vi "Simulation-07.vi"() -> ()   [LabVIEW 2020]
uses:
  librarian_class/typedefs/book_state--enum.ctl
  shared/request--enum.ctl
  librarian_class/librarian.lvclass
  client_class/client.lvclass
panel:
  out "success":bool
  out "lib error out":errorcluster
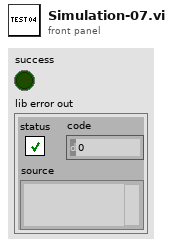
[diagram p1: front panel]
types:
  T1 = typedef "request--enum.ctl" = enum16{"CHECKIN", "CHECKOUT"}
  T2 = typedef "librarian.lvclass/book_state--enum.ctl" = enum16{"CHECKEDIN", "CHECKEDOUT", "DAMAGED"}
  T3 = typedef "message--cluster.ctl" = cluster{"header":string, "cmd":T1, "title":string, "book":string}
  T4 = typedef "librarian.lvclass/lib_map_value--cluster.ctl" = cluster{"book state":T2, "text":string, "hash":string}
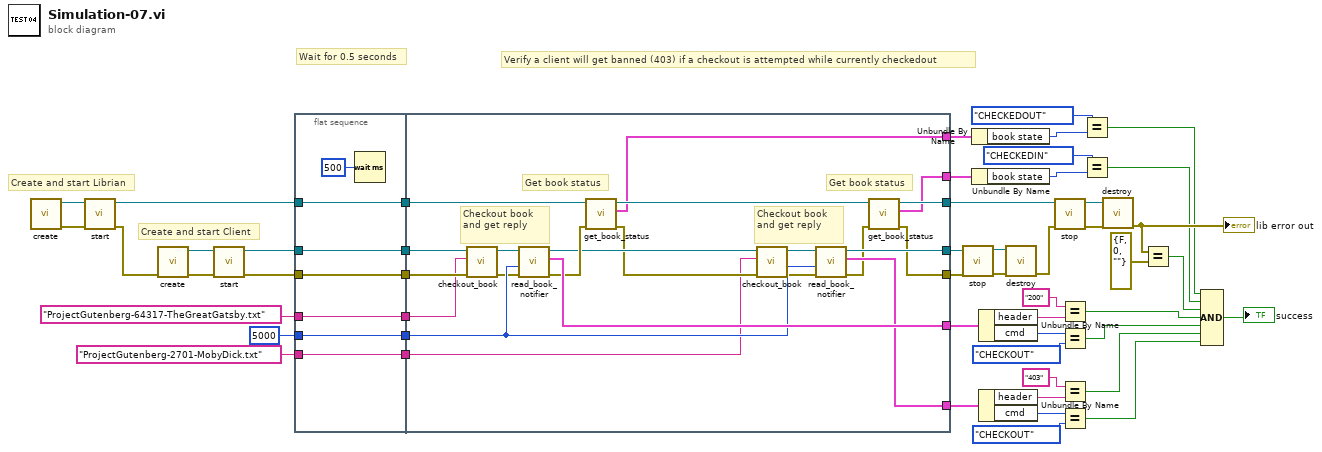
[diagram p0: block diagram]
diagram:
  # "Verify a client will get banned (403) if a checkout is attempted while currently checkedout"
  # "Wait for 0.5 seconds"
  # "Create and start Client"
  # "Create and start Librian"
  n1 = call "create.vi"() -> ("error out"=w50:errorcluster, "librarian_sm out"=w51:refnum<class "librarian.lvclass">)  [unwired: 10 in]
  n2 = call "start.vi"("error in (no error)"=w50, "librarian_sm in"=w51) -> ("error out"=w30:errorcluster, "librarian_sm out"=w41:refnum<class "librarian.lvclass">)  [unwired: 8 in]
  n3 = call "create.vi"("error in (no error)"=w30) -> ("error out"=w46:errorcluster, "librarian_sm out"=w47:refnum<class "client.lvclass">)  [unwired: 9 in]
  n4 = call "start.vi"("error in (no error)"=w46, "librarian_sm in"=w47) -> ("error out"=w43:errorcluster, "librarian_sm out"=w42:refnum<class "client.lvclass">)  [unwired: 8 in]
  n5 = flat-sequence {
    tunnel: "ProjectGutenberg-64317-TheGreatGatsby.txt" ("book title") -> [w53]
    tunnel: 5000 ("timeout in ms (-1)") -> [w56]
    tunnel: w41 -> [w57]
    tunnel: w42 -> [w58]
    tunnel: w43 -> [w54]
    tunnel: [w54] -> w35
    tunnel: [w58] -> w34
    tunnel: [w57] -> w33
    tunnel: [w56] -> w32
    tunnel: [w53] -> w31
    tunnel: [w52] -> w2
    tunnel: "ProjectGutenberg-2701-MobyDick.txt" ("book title") -> [w52]
    tunnel: [w80] -> w14
    tunnel: [w67] -> w38
    tunnel: [w78] -> w39
    tunnel: [w70] -> w40
    tunnel: [w77] -> w13
    tunnel: w31 -> [w61]
    tunnel: w32 -> [w79]
    tunnel: w33 -> [w72]
    tunnel: w34 -> [w75]
    tunnel: w35 -> [w76]
    tunnel: [w66] -> w23
    tunnel: [w65] -> w24
    tunnel: w2 -> [w59]
    frame #0 {
      n6 = Wait (ms)(milliseconds to wait=u32 500) -> ()  [unwired: 1 out]
    }
    frame #1 {
      # "Get book status"
      # "Get book status"
      # "Checkout book and get reply"
      # "Checkout book and get reply"
      n7 = call "checkout_book.vi"("error in (no error)"=w76, "book title"=w61, "client in"=w75) -> ("error out"=w73:errorcluster, "client out"=w74:refnum<class "client.lvclass">)  [unwired: 7 in]
      n8 = call "read_book_notifier.vi"("error in (no error)"=w73, "timeout in ms (-1)"=w79, "client in"=w74) -> ("error out"=w69:errorcluster, "msg"=w80:T3, "client out"=w62:refnum<class "client.lvclass">)  [unwired: 6 in]
      n9 = call "get_book_status.vi"("error in (no error)"=w69, "librarian in"=w72) -> ("error out"=w60:errorcluster, "book status"=w65:T4, "librarian out"=w71:refnum<class "librarian.lvclass">)  [unwired: 7 in]
      n10 = call "checkout_book.vi"("error in (no error)"=w60, "book title"=w59, "client in"=w62) -> ("error out"=w64:errorcluster, "client out"=w63:refnum<class "client.lvclass">)  [unwired: 7 in]
      n11 = call "read_book_notifier.vi"("error in (no error)"=w64, "timeout in ms (-1)"=w79, "client in"=w63) -> ("error out"=w68:errorcluster, "msg"=w77:T3, "client out"=w78:refnum<class "client.lvclass">)  [unwired: 6 in]
      n12 = call "get_book_status.vi"("error in (no error)"=w68, "librarian in"=w71) -> ("error out"=w67:errorcluster, "book status"=w66:T4, "librarian out"=w70:refnum<class "librarian.lvclass">)  [unwired: 7 in]
    }
  }
  n13 = call "stop.vi"("error in (no error)"=w38, "librarian_sm in"=w39) -> ("error out"=w44:errorcluster, "librarian_sm out"=w45:refnum<class "client.lvclass">)  [unwired: 8 in]
  n14 = Unbundle By Name(w24) -> ("book state"=w28:T2)
  n15 = Unbundle By Name(w23) -> ("book state"=w25:T2)
  n16 = Unbundle By Name(w14) -> ("header"=w22:string, "cmd"=w20:T1)
  n17 = Unbundle By Name(w13) -> ("header"=w15:string, "cmd"=w17:T1)
  n18 = call "destroy.vi"("error in (no error)"=w44, "librarian_sm in"=w45) -> ("error out"=w29:errorcluster)  [unwired: 8 in, 1 out]
  n19 = call "stop.vi"("error in (no error)"=w29, "librarian_sm in"=w40) -> ("error out"=w48:errorcluster, "librarian_sm out"=w49:refnum<class "librarian.lvclass">)  [unwired: 8 in]
  n20 = Equal?(x="200", y=w22) -> (x = y?=w7:bool)
  n21 = Equal?(x=w20, y=request--enum."CHECKOUT") -> (x = y?=w6:bool)
  n22 = Equal?(x="403", y=w15) -> (x = y?=w5:bool)
  n23 = Equal?(x=w17, y=request--enum."CHECKOUT") -> (x = y?=w4:bool)
  n24 = Equal?(x=book_state--enum."CHECKEDOUT", y=w28) -> (x = y?=w10:bool)
  n25 = Equal?(x=book_state--enum."CHECKEDIN", y=w25) -> (x = y?=w9:bool)
  n26 = call "destroy.vi"("error in (no error)"=w48, "librarian_sm in"=w49) -> ("error out"=w11:errorcluster)  [unwired: 8 in, 1 out]
  "lib error out" <- w11
  n27 = Equal?(x=w11, y=errorcluster {"status"=FALSE, "code"=0, "source"=""}) -> (x = y?=w8:bool)
  n28 = Compound Arithmetic op=AND(w10, w9, w8, w7, w6, w5, w4) -> (→"success":bool)
